vi "Render Unescaped Tag with Hook.vi"(8 "Error In":errorcluster) -> (0 "Error Out":errorcluster)   [LabVIEW 2018, in "Tests.lvlib" / "Render.lvlib"]
uses:
  Render.lvlib
  Support/Mock Render Variable Hook/Mock Render Variable Hook.lvclass
  D:/Users/cfield/Code/Field R&D Services/Labstache/src/Toolkit/Hooks/Pre-Render Variable/Render Variable.lvclass
  src/Toolkit/Hooks/Pre-Render Variable/Render Variable.lvclass
  src/Toolkit/Data/Map/Map.lvclass
  D:/Users/cfield/Code/Field R&D Services/Labstache/src/Toolkit/Data/Datum/Datum.lvclass
  src/Toolkit/Low-Level/Support/Lex String.vi
  src/Toolkit/Data/Map/Support/From String.vi
  src/Toolkit/Low-Level/Support/Render to String.vi
  <vilib>/addons/_JKI Toolkits/Caraya/classes/Test/Test.lvclass
  <vilib>/addons/_JKI Toolkits/Caraya/classes/Assert/Assert.lvclass
  src/Toolkit/Toolkit.lvlib
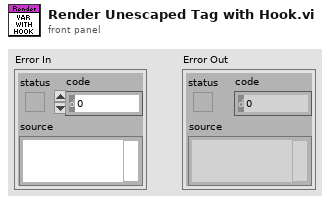
[diagram p1: front panel]
types:
  T1 = cluster{"Render":cluster{"Variable":refnum<class "Render Variable.lvclass">}}
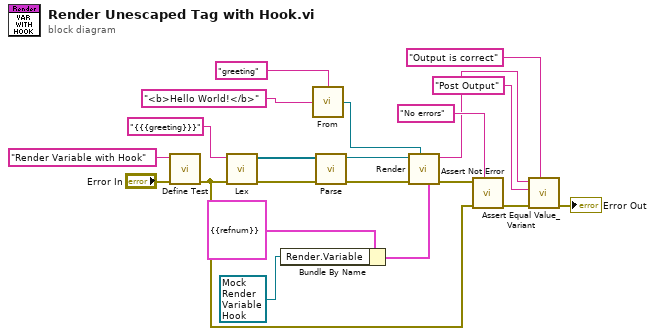
[diagram p0: block diagram]
diagram:
  n1 = call <vilib>:"Define Test.vi"("error in (no error)"="Error In", "Label (VI Title)"="Render Variable with Hook") -> ("error out"=w4:errorcluster)  [unwired: 9 in]
  n2 = call-poly "Lex.vi"("Error In"=w4, "Input"="{{{greeting}}}" ("format string")) -> ("Error Out"=w13:errorcluster, "Tokens"=w11:refnum<class "Token.lvclass">[])  [unwired: 8 in]
  n3 = Bundle By Name(cluster=T1 {"Render"={"Variable"=refnum}} ("Hooks"), "Render.Variable"=refnum<class "Mock Render Variable Hook.lvclass"> refnum ("Tests.lvlib:Render.lvlib:Mock Render Variable Hook.lvclass")) -> (w2:T1)
  n4 = call-poly "From.vi"("Value"="<b>Hello World!</b>", "Key"="greeting") -> ("Map"=w5:refnum<class "Map.lvclass">)
  n5 = call "Parse.vi"("Error In"=w13, "Tokens"=w11) -> ("Error Out"=w10:errorcluster, "Abstract Syntax Tree"=w9:refnum<class "Root.lvclass">)  [unwired: 8 in]
  n6 = call-poly "Render.vi"("Hooks"=w2, "Data"=w5, "Error In"=w10, "Abstract Syntax Tree"=w9) -> ("Error Out"=w15:errorcluster, "Output"=w8:string)  [unwired: 6 in]
  n7 = call <vilib>:"Assert Not Error.vi"("Label"="No errors", "error in (no error)"=w4, "Not Error?"=w15) -> ("error out"=w18:errorcluster)  [unwired: 8 in]
  n8 = call <vilib>:"Assert Equal Value_Variant.vi"("Label"="Output is correct", "error in (no error)"=w18, "Y"="Post Output" ("Value"), "X"=w8) -> ("error out"=→"Error Out":errorcluster)  [unwired: 7 in]
